vi "GetVision.vi"   [LabVIEW 2018]
uses:
  <vilib>/Rock Robotics/Network Tables/NT Read Number.vi
  SensorReadings.vi
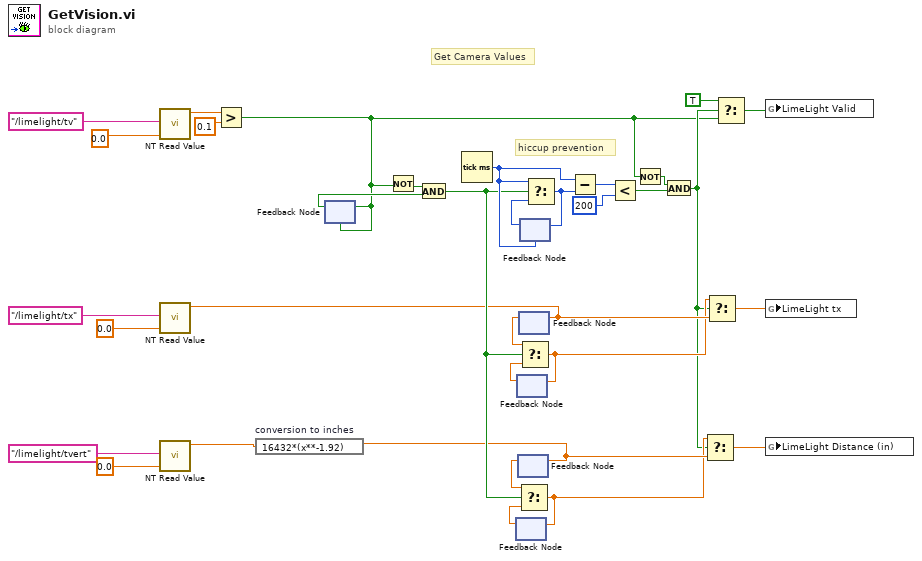
[diagram p0: block diagram]
diagram:
  # "hiccup prevention"
  # "Get Camera Values"
  n1 = call-poly <vilib>:"NT Read Value.vi"("Default Value"=0.0, "Name"="/limelight/tv") -> ("Numeric"=w26:dbl)  [unwired: 8 in, 1 out]
  n2 = call-poly <vilib>:"NT Read Value.vi"("Default Value"=0.0, "Name"="/limelight/tx") -> ("Numeric"=w8:dbl)  [unwired: 8 in, 1 out]
  n3 = call-poly <vilib>:"NT Read Value.vi"("Default Value"=0.0, "Name"="/limelight/tvert") -> ("Numeric"=w28:dbl)  [unwired: 8 in, 1 out]
  n4 = Greater?(x=w26, y=0.1) -> (0:w1:bool)
  n5 = expression code="16432*(x**-1.92)" "conversion to inches"(w28) -> (w10:dbl)
  n6 = feedback-in #1(w1) -> ()
  n7 = feedback #1(w1) -> (w24:bool)
  n8 = Not(x=w1) -> (.not. x?=w23:bool)
  n9 = And(x=w23, y=w24) -> (x .and. y?=w13:bool)
  n10 = Tick Count (ms)() -> (millisecond timer value=w20:u32)
  n11 = feedback #2() -> (w15:dbl)  [unwired: 1 in]
  n12 = feedback #3() -> (w17:dbl)  [unwired: 1 in]
  n13 = feedback #4() -> (w14:dbl)  [unwired: 1 in]
  n14 = feedback-in #4(w10) -> ()
  n15 = feedback-in #5(w8) -> ()
  n16 = feedback #5() -> (w16:dbl)  [unwired: 1 in]
  n17 = Select(t=w14, s=w13, f=w15) -> (s? t:f=w9:dbl)
  n18 = feedback-in #2(w9) -> ()
  n19 = feedback #6(w20) -> (w22:u32)
  n20 = Select(t=w16, s=w13, f=w17) -> (s? t:f=w7:dbl)
  n21 = feedback-in #3(w7) -> ()
  n22 = Select(t=w20, s=w13, f=w22) -> (s? t:f=w21:u32)
  n23 = feedback-in #6(w21) -> ()
  n24 = Subtract(x=w20, y=w21) -> (x-y=w19:u32)
  n25 = Less?(x=w19, y=u32 200) -> (x < y?=w4:bool)
  n26 = Not(x=w1) -> (.not. x?=w2:bool)
  n27 = And(x=w2, y=w4) -> (x .and. y?=w3:bool)
  n28 = Select(t=w9, s=w3, f=w10) -> (s? t:f=w11:dbl)
  n29 = Select(t=w7, s=w3, f=w8) -> (s? t:f=w12:dbl)
  n30 = Select(t=TRUE, s=w3, f=w1) -> (s? t:f=w5:bool)
  n31 = global write "SensorReadings.vi" "LimeLight Valid"(w5) -> ()
  n32 = global write "SensorReadings.vi" "LimeLight tx"(w12) -> ()
  n33 = global write "SensorReadings.vi" "LimeLight Distance (in)"(w11) -> ()
